vi "QR Get Queue .vi"(8 "error in (no error)":errorcluster, 11 "Name":string) -> (0 "error out":errorcluster, 3 "Queue Out":T1)   [LabVIEW 2013, in "AMC.lvlib"]
doc: "This VI removes the host connection from the connection manager list if it becomes disconnected for any reason."
uses:
  AMC.lvlib
  _SubVIs/TypeDefs/Message Queue.ctl
  _SubVIs/TypeDefs/Message.ctl
  Keyed Array/KeyedArray.ctl
  _TypeDefs/QueueRegistryMethod.ctl
  _TypeDefs/QueueRegistryProperties.ctl
  Keyed Array/Tools_KeyedArray.lvlib
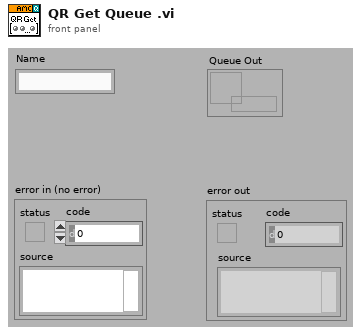
[diagram p1: front panel]
types:
  T1 = typedef "AMC.lvlib/Message Queue.ctl" = refnum<queue>
  T2 = typedef "AMC.lvlib/QueueRegistryProperties.ctl" = cluster{"Name":string}
  T3 = typedef "AMC.lvlib/QueueRegistryMethod.ctl" = enum16{"Initialize", "Add Queue", "Set Properties", "Get Queue by Index", "Get Queue by Name", "Remove Queue", "Remove All Queues"}
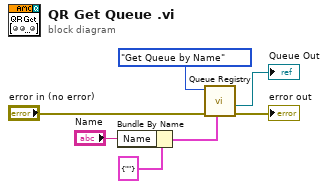
[diagram p0: block diagram]
diagram:
  n1 = Bundle By Name(cluster=T2 {"Name"=""} ("Properties In"), "Name"="Name") -> (w4:T2)
  n2 = call "Queue Registry.vi"("Properties in"=w4, "error in (no error)"="error in (no error)", "Method"=QueueRegistryMethod."Get Queue by Name") -> ("error out"=→"error out":errorcluster, "Message Queue out"=→"Queue Out":T1)  [unwired: 2 in, 5 out]
